vi "SI string to double.vi"(8 "error in":errorcluster, 11 "SI String":string="60.2dA") -> (0 "error out":errorcluster, 1 "after match":string, 2 "before match":string, 3 "Numeric output":dbl)   [LabVIEW 2018]
uses:
  <vilib>/regexp/Match Regular Expression.xnode
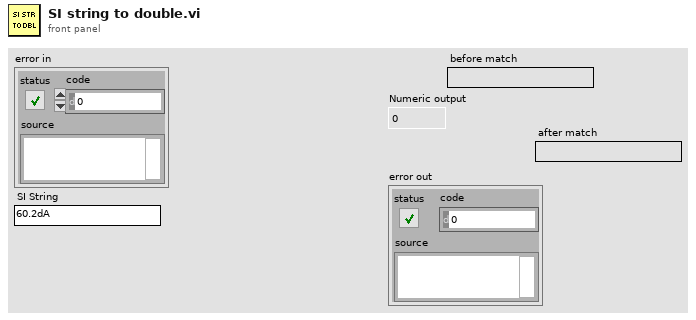
[diagram p1: front panel]
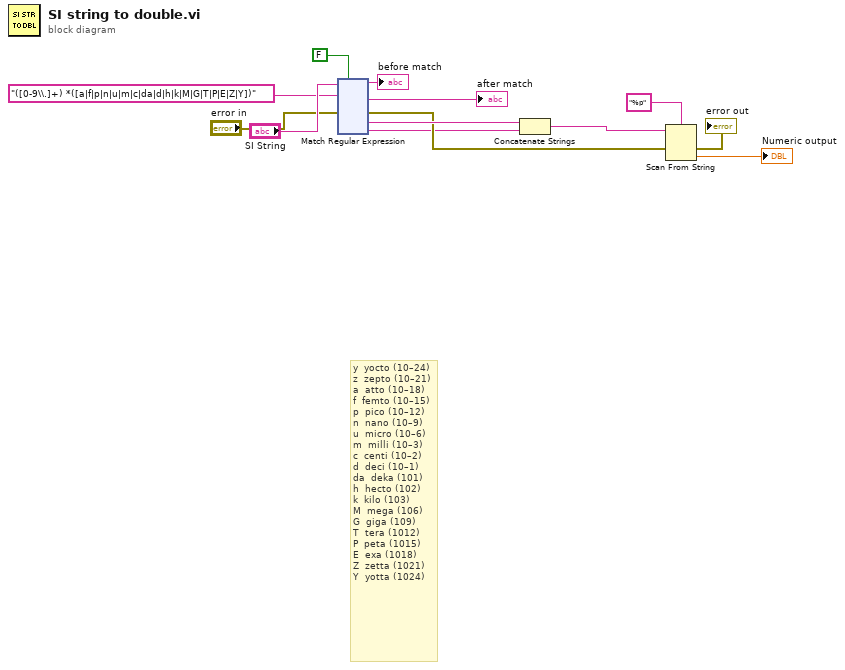
[diagram p0: block diagram]
diagram:
  # "y \tyocto (10–24)\nz \tzepto (10–21)\na \tatto (10–18)\nf \tfemto (10–15)\np \tpico (10–12)\nn \tnano (10–9)\nu \tmicro (10–6)\nm \tmilli (10–3)\nc \tcenti (10–2)\nd \tdeci (10–1)\nda \tdeka (101)\nh \thecto (102)\nk \tkilo (103)\nM \tmega (106)\nG \tgiga (109)\nT \ttera (1012)\nP \tpeta (1015)\nE \texa (1018)\nZ \tzetta (1021)\nY \tyotta (1024)"
  n1 = xnode "Match Regular Expression"("input string"="SI String", "regular expression"="([0-9\\.]+) *([a|f|p|n|u|m|c|da|d|h|k|M|G|T|P|E|Z|Y])" ("source"), "error in"="error in", "ignore case? (F)"=FALSE) -> ("before match"=→"before match":string, "after match"=→"after match":string, "error out"=w6:errorcluster, "submatch 1"=w8:string, "submatch 2"=w3:string)  [unwired: 2 in, 2 out]
  n2 = Concatenate Strings(w8, w3) -> (w9:string)
  n3 = Scan From String(format string="%p" ("source"), input string=w9, error in=w6) -> (error out=→"error out":errorcluster, output 1=→"Numeric output":dbl)  [unwired: 2 in, 2 out]
